vi "Reproductorc.vi"() -> ()   [LabVIEW 2017]
uses:
  <vilib>/sound2/lvsound2.llb/Sound File Position.ctl
  <vilib>/sound2/lvsound2.llb/Sound File Read (DBL).vi
  <vilib>/measure/maspectr.llb/FFT Spectrum (Mag-Phase) for N Chan.vi
  <vilib>/sound2/lvsound2.llb/Sound Output Write (DBL).vi
  <vilib>/measure/NI_MAPro.lvlib
panel:
  out "Cancion":waveform(dbl)[](graph)
  out "FFT":cluster{"f0":dbl, "df":dbl, "magnitude":dbl[]}[](graph)
  out "Array":path[](array[path])
  out "filenames":string[](array[string])
  in  "Skip Forward Button":bool
  in  "Skip Back Button":bool
  in  "Seek Forward Button":bool
  in  "Seek Back Button":bool
  in  "Media Stop Button":bool
  in  "Pause Button":bool
  in  "Play Button":bool
  in  "stop":bool
  in  "path":path
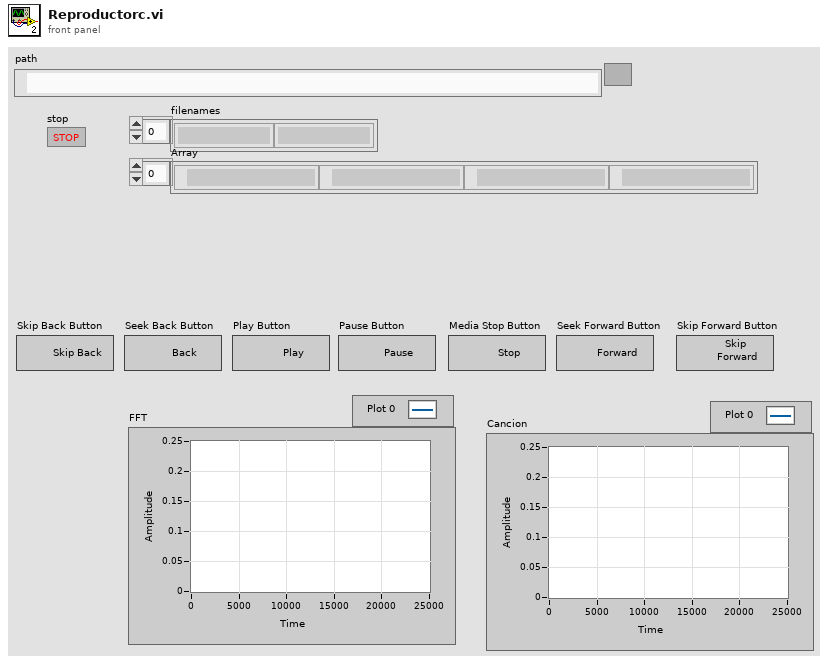
[diagram p1: front panel]
types:
  T1 = typedef "Sound Output Task ID.ctl" = u32
  T2 = typedef "Sound File Refnum.ctl" = refnum<file>
  T3 = cluster{"sound file refnum out":T2, "Error_A":errorcluster, "task ID out":T1, "Error_B":errorcluster, "Indice":i32, "Reproduccion":i32, "Numero de Cancion":i32}
  T4 = typedef "Sound File Position.ctl" = u16
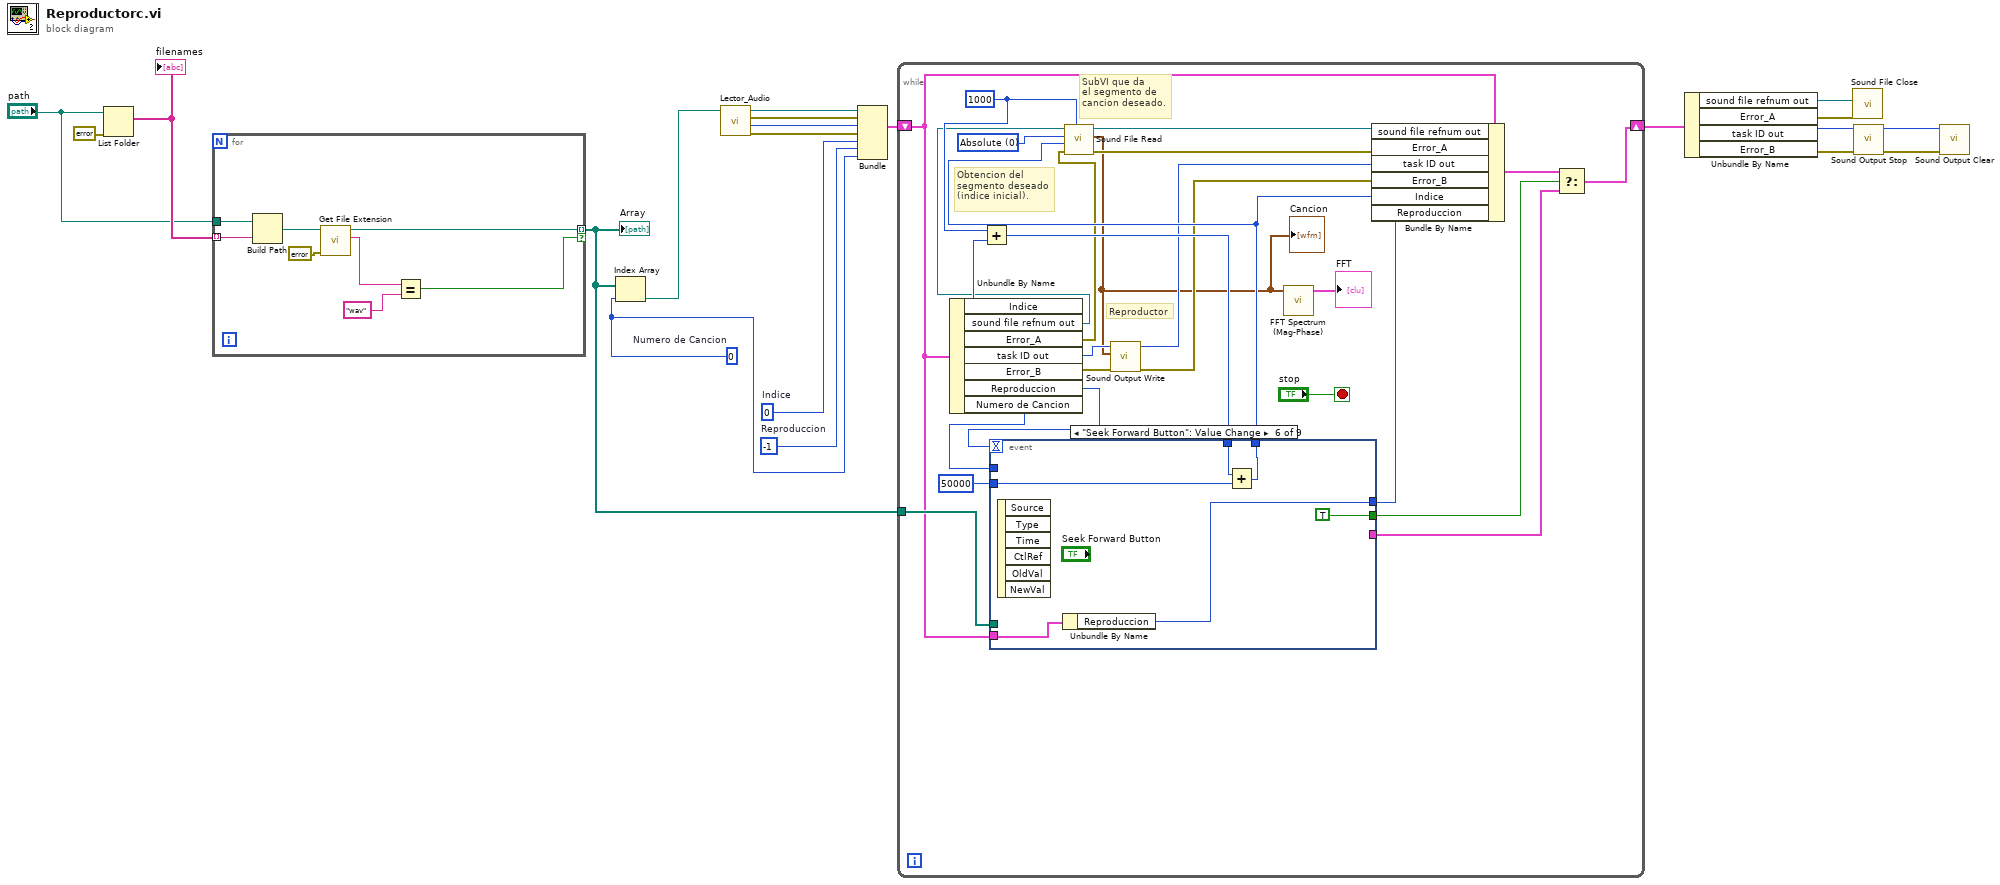
[diagram p0: block diagram]
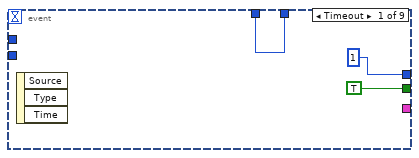
[diagram p2: hidden frame]
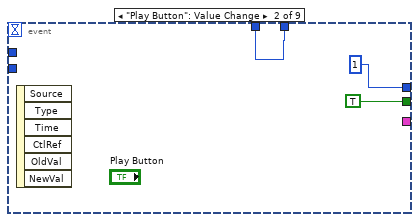
[diagram p3: hidden frame]
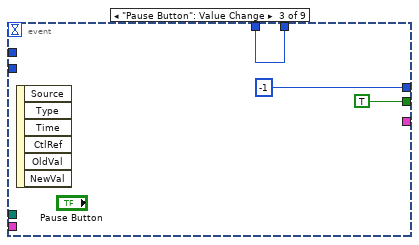
[diagram p4: hidden frame]
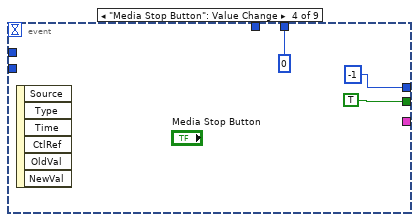
[diagram p5: hidden frame]
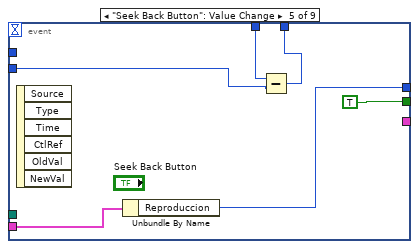
[diagram p6: hidden frame]
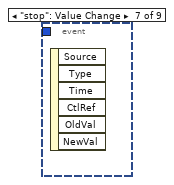
[diagram p7: hidden frame]
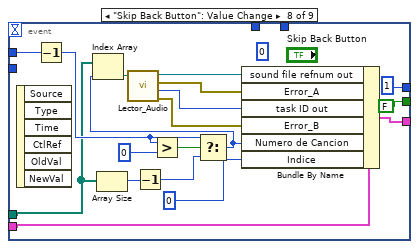
[diagram p8: hidden frame]
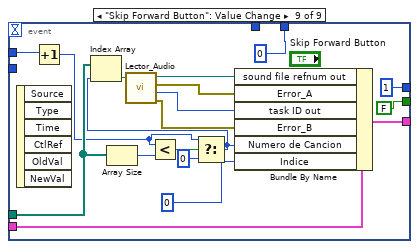
[diagram p9: hidden frame]
diagram:
  w7 = 0  # Numero de Cancion
  w11 = -1  # Reproduccion
  w12 = 0  # Indice
  n1 = List Folder(path="path", error in=errorcluster {"status"=FALSE, "code"=0, "source"=""}) -> (filenames=w9:string[])  [unwired: 2 in, 3 out]
  "filenames" <- w9
  n2 = for {
    tunnel: w9 -> [w28] mode=indexing
    tunnel: "path" -> [w27]
    tunnel: [w22] -> w6 mode=indexing if=w21
    n3 = Build Path(base path=w27, name or relative path=w28) -> (appended path=w26:path)
    n4 = call <vilib>:"Get File Extension.vi"("error in (no error)"=errorcluster {"status"=FALSE, "code"=0, "source"=""}, "file"=w26) -> ("lowercase file extension"=w24:string, "dup file"=w22:path)  [unwired: 5 in, 3 out]
    n5 = Equal?(x=w24, y="wav") -> (x = y?=w21:bool)
  }
  "Array" <- w6
  n6 = Index Array "Index Array"(array=w6, index=w7) -> (element=w5:path)
  n7 = call "Lector_Audio.vi"("path"=w5) -> ("Error_B"=w1:errorcluster, "task ID out"=w2:T1, "Error_A"=w3:errorcluster, "sound file refnum out"=w4:T2)  [unwired: 7 in]
  n8 = Bundle("sound file refnum out"=w4, "Error_A"=w3, "task ID out"=w2, "Error_B"=w1, "Indice"=w12, "Reproduccion"=w11, "Numero de Cancion"=w7) -> (w18:T3)  [unwired: 1 in]
  n9 = while {
    shift-right: [w35] -> w17
    shift-left: w18 -> [w34]
    tunnel: w6 -> [w44]
    stop <- "stop" stop-if-true
    w51 = 1000 ("number of samples/ch (-1: all)")
    w54 = T4 0 items=["Absolute"=0, "Relative"=2] ("position mode")
    # "SubVI que da\nel segmento de\ncancion deseado."
    # "Reproductor"
    # "Obtencion del \nsegmento deseado\n(indice inicial)."
    n10 = Unbundle By Name(w34) -> ("Indice"=w52:i32, "sound file refnum out"=w41:T2, "Error_A"=w40:errorcluster, "task ID out"=w42:T1, "Error_B"=w43:errorcluster, "Reproduccion"=w47:i32, "Numero de Cancion"=w45:i32)
    n11 = Add(x=w51, y=w52) -> (x+y=w50:i32)
    n12 = event shown="[5] \"Seek Forward Button\": Value Change" {
      selector: _ -> [_ _ _ _ _ _ _ _ _]
      dyn-events: _ -> [_ _ _ _ _ _ _ _ _]
      timeout: w47 -> [_ _ _ _ _ _ _ _ _]
      tunnel: w50 -> [w57 w59 w62 _ w72 w77 _ _ _]
      tunnel: [w57 w59 w62 0 w71 w76 _ _ 0] -> w49
      tunnel: [1 1 -1 -1 w67 w73 _ 1 1] -> w48
      tunnel: 50000 ("y") -> [_ _ _ _ w70 w78 _ _ _]
      tunnel: w45 -> [_ _ _ _ _ _ _ w83 w114]
      tunnel: w44 -> [_ _ _ _ _ _ _ w81 w103]
      tunnel: w34 -> [_ _ _ _ w68 w74 _ w87 w112]
      tunnel: [_ _ _ _ _ _ _ w86 w106] -> w33
      tunnel: [TRUE TRUE TRUE TRUE TRUE TRUE _ FALSE FALSE] -> w32
      event Timeout {
        n13 = event-data() -> ()  [unwired: 1 in, 3 out]
      }
      event "Play Button": Value Change {
        n14 = event-data() -> ()  [unwired: 1 in, 6 out]
      }
      event "Pause Button": Value Change {
        n15 = event-data() -> ()  [unwired: 1 in, 6 out]
      }
      event "Media Stop Button": Value Change {
        n16 = event-data() -> ()  [unwired: 1 in, 6 out]
      }
      event "Seek Back Button": Value Change {
        n17 = event-data() -> ()  [unwired: 1 in, 6 out]
        n18 = Unbundle By Name(w68) -> ("Reproduccion"=w67:i32)
        n19 = Subtract(x=w72, y=w70) -> (x-y=w71:i32)
      }
      event "Seek Forward Button": Value Change {
        n20 = event-data() -> ()  [unwired: 1 in, 6 out]
        n21 = Unbundle By Name(w74) -> ("Reproduccion"=w73:i32)
        n22 = Add(x=w77, y=w78) -> (x+y=w76:i32)
      }
      event "stop": Value Change {
        n23 = event-data() -> ()  [unwired: 1 in, 6 out]
      }
      event "Skip Back Button": Value Change {
        (unwired) 0
        n24 = event-data() -> ()  [unwired: 1 in, 6 out]
        n25 = Decrement(x=w83) -> (x-1=w90:i32)
        n26 = Array Size(array=w81) -> (size(s)=w80:i32)
        n27 = Decrement(x=w80) -> (x-1=w79:i32)
        n28 = Greater?(x=w90, y=0 ("f")) -> (0:w91:bool)
        n29 = Select(t=w90, s=w91, f=w79) -> (s? t:f=w89:i32)
        n30 = Index Array(array=w81, index=w89) -> (element=w96:path)
        n31 = call "Lector_Audio.vi"("path"=w96) -> ("Error_B"=w92:errorcluster, "task ID out"=w93:T1, "Error_A"=w94:errorcluster, "sound file refnum out"=w95:T2)  [unwired: 7 in]
        n32 = Bundle By Name(cluster=w87, "sound file refnum out"=w95, "Error_A"=w94, "task ID out"=w93, "Error_B"=w92, "Numero de Cancion"=w89, "Indice"=0) -> (w86:T3)
      }
      event "Skip Forward Button": Value Change {
        n33 = event-data() -> ()  [unwired: 1 in, 6 out]
        n34 = Increment(x=w114) -> (x+1=w100:i32)
        n35 = Array Size(array=w103) -> (size(s)=w102:i32)
        n36 = Less?(x=w100, y=w102) -> (x < y?=w101:bool)
        n37 = Select(t=w100, s=w101, f=0) -> (s? t:f=w98:i32)
        n38 = Index Array(array=w103, index=w98) -> (element=w113:path)
        n39 = call "Lector_Audio.vi"("path"=w113) -> ("Error_B"=w108:errorcluster, "task ID out"=w109:T1, "Error_A"=w110:errorcluster, "sound file refnum out"=w111:T2)  [unwired: 7 in]
        n40 = Bundle By Name(cluster=w112, "sound file refnum out"=w111, "Error_A"=w110, "task ID out"=w109, "Error_B"=w108, "Numero de Cancion"=w98, "Indice"=0) -> (w106:T3)
      }
    }
    n41 = call-poly <vilib>:"Sound File Read.vi"("number of samples/ch (-1: all)"=w51, "error in (no error)"=w40, "position offset"=w49, "position mode"=w54, "sound file refnum"=w41) -> ("error out"=w39:errorcluster, "data"=w29:waveform(dbl)[], "sound file refnum out"=w31:T2)  [unwired: 2 in, 2 out]
    "Cancion" <- w29
    n42 = call-poly <vilib>:"Sound Output Write.vi"("error in (no error)"=w43, "data"=w29, "task ID"=w42) -> ("error out"=w37:errorcluster, "task ID out"=w38:T1)  [unwired: 7 in]
    n43 = call-poly <vilib>:"FFT Spectrum (Mag-Phase).vi"("time signals"=w29) -> ("magnitudes"=→"FFT":cluster{"f0":dbl, "df":dbl, "magnitude":dbl[]}[])  [unwired: 6 in, 4 out]
    n44 = Bundle By Name(cluster=w34, "sound file refnum out"=w31, "Error_A"=w39, "task ID out"=w38, "Error_B"=w37, "Indice"=w49, "Reproduccion"=w48) -> (w36:T3)
    n45 = Select(t=w36, s=w32, f=w33) -> (s? t:f=w35:T3)
  }
  n46 = Unbundle By Name(w17) -> ("sound file refnum out"=w16:T2, "Error_A"=w15:errorcluster, "task ID out"=w14:T1, "Error_B"=w13:errorcluster)
  n47 = call <vilib>:"Sound File Close.vi"("error in (no error)"=w15, "sound file refnum"=w16) -> ()  [unwired: 9 in, 1 out]
  n48 = call <vilib>:"Sound Output Stop.vi"("error in (no error)"=w13, "task ID"=w14) -> ("error out"=w19:errorcluster, "task ID out"=w20:T1)  [unwired: 8 in]
  n49 = call <vilib>:"Sound Output Clear.vi"("error in (no error)"=w19, "task ID"=w20) -> ()  [unwired: 9 in, 1 out]
